vi "delete Segment.vi"(8 "error in (no error)":errorcluster caption="Fehler (Eingang, kein Fehler)", 10 "Index":i32, 11 "Test Eingang":refnum<class "Test.lvclass"> caption="DNL_LabVIEW Object in") -> (0 "error out":errorcluster caption="Fehler (Ausgang)", 3 "Test Ausgang":refnum<class "Test.lvclass"> caption="DNL_LabVIEW Object out")   [LabVIEW 2013, in "DatenKlassen.lvlib" / "Test.lvclass"]
uses:
  Test.lvclass
  Test.lvclass/Test.ctl
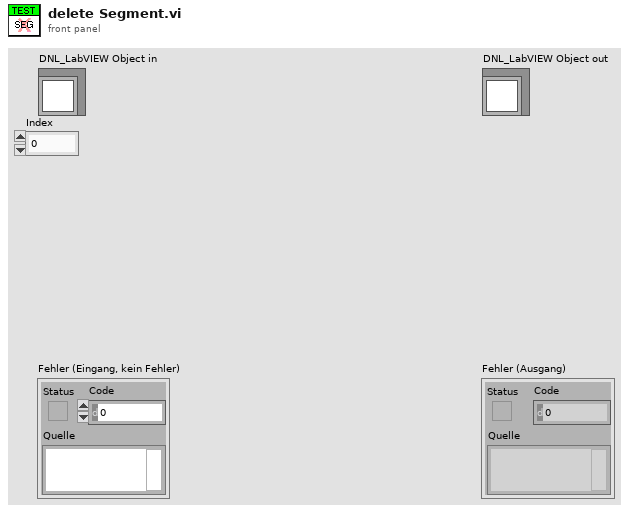
[diagram p1: front panel]
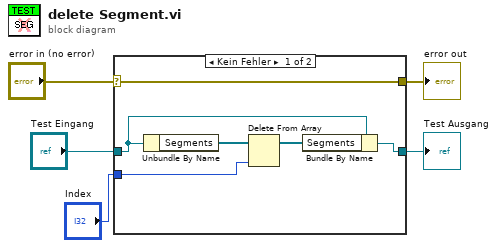
[diagram p0: block diagram]
diagram:
  n1 = case shown="Kein Fehler" "error in (no error)" {
    selector: "error in (no error)" -> [w11 w13]
    tunnel: [w11 w13] -> w4
    tunnel: [w7 w12] -> w2
    tunnel: "Test Eingang" -> [w9 w12]
    tunnel: "Index" -> [w6 _]
    frame No Error {
      n2 = Unbundle By Name(w9) -> ("Segments"=w10:refnum<class "Segment.lvclass">[])
      n3 = Delete From Array(array=w10, index=w6) -> (array with subset deleted=w8:refnum<class "Segment.lvclass">[])  [unwired: 1 in, 1 out]
      n4 = Bundle By Name(cluster=w9, "Segments"=w8) -> (w7:refnum<class "Test.lvclass">)
    }
    frame Error {
    }
  }
  "error out" <- w4
  "Test Ausgang" <- w2
